vi "IPC-Core-ModbusModule.vi"(8 "error in":errorcluster, 9 "ErrorQRef":refnum<queue>, 10 "ModbusQRef":refnum<queue>, 11 "CmdQRef":refnum<queue>) -> (0 "error out":errorcluster)   [LabVIEW 2014]
uses:
  Configuration-Global.vi
panel:
  out "Modbus停止响应器":refnum<notifier>
  out "Modbus停止通知器":refnum<notifier>
  out "Modbus开始响应器":refnum<notifier>
  out "Modbus开始通知器":refnum<notifier>
  out "Modbus Deamo is Running":bool
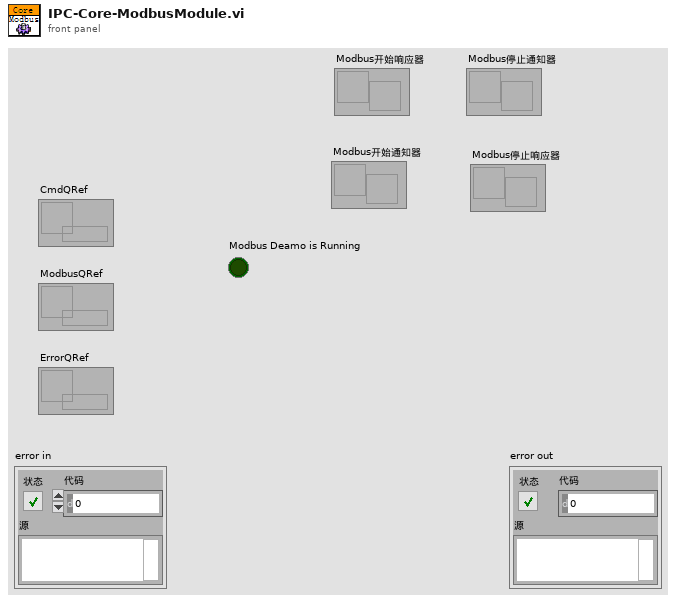
[diagram p1: front panel]
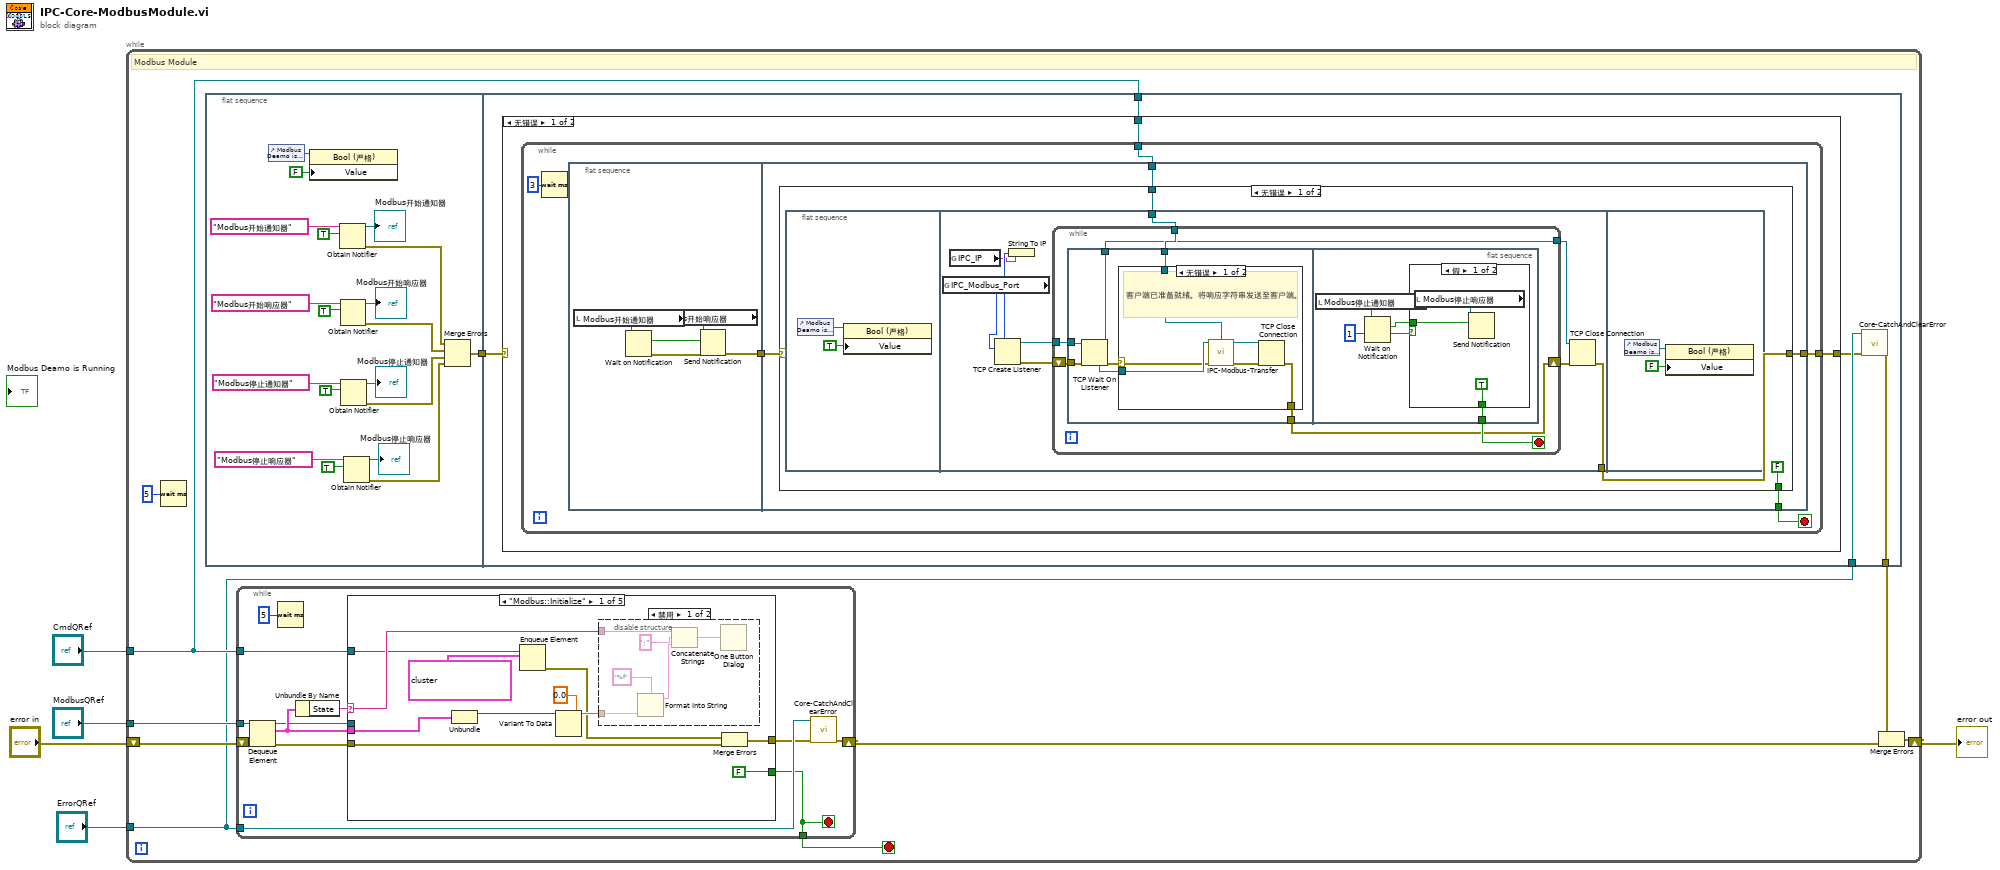
[diagram p0: block diagram]
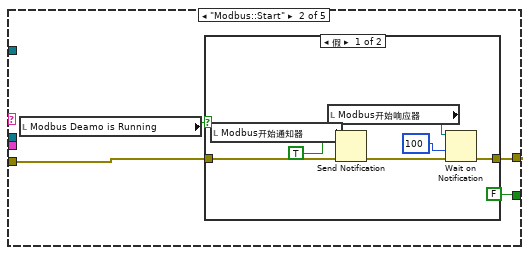
[diagram p3: hidden frame]
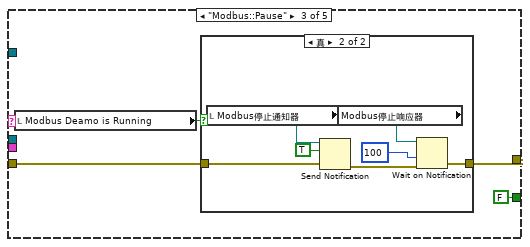
[diagram p5: hidden frame]
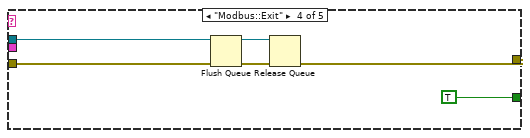
[diagram p7: hidden frame]
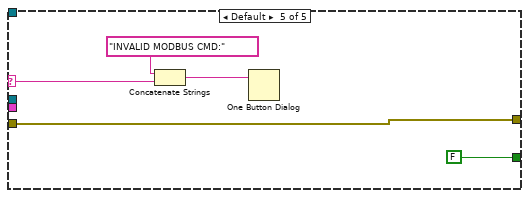
[diagram p8: hidden frame]
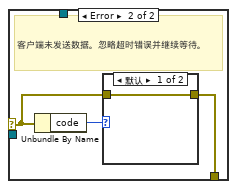
[diagram p9: hidden frame]
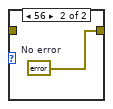
[diagram p10: hidden frame]
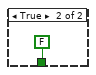
[diagram p11: hidden frame]
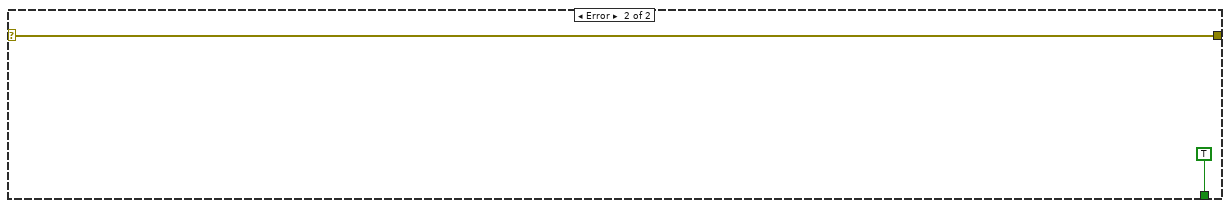
[diagram p12: hidden frame]
diagram:
  n1 = while {
    shift-right: [w6] -> w2
    shift-left: "error in" -> [w10]
    tunnel: "ErrorQRef" -> [w9]
    tunnel: "ModbusQRef" -> [w14]
    tunnel: "CmdQRef" -> [w11]
    stop <- w13 stop-if-true
    # "Modbus Module"
    n2 = Wait (ms)(milliseconds to wait=u32 5 ("等待时间（毫秒）")) -> ()  [unwired: 1 out]
    n3 = flat-sequence {
      tunnel: [w80] -> w12
      tunnel: w12 -> [w103]
      tunnel: w11 -> [w102]
      tunnel: w9 -> [w101]
      tunnel: [w99] -> w7
      frame #0 {
        n4 = control-ref of="Modbus Deamo is Running"() -> (w97:refnum<vi>)
        n5 = property class="Bool (严格)"(reference=w97, "Value"=FALSE ("值")) -> ()  [unwired: 1 in, 2 out]
        n6 = Obtain Notifier(name (unnamed)="Modbus开始通知器" ("名称（未命名）"), notification data type=TRUE) -> (notifier out=→"Modbus开始通知器":refnum<notifier>, error out=w84:errorcluster)  [unwired: 2 in, 1 out]
        n7 = Obtain Notifier(name (unnamed)="Modbus开始响应器" ("名称（未命名）"), notification data type=TRUE) -> (notifier out=→"Modbus开始响应器":refnum<notifier>, error out=w83:errorcluster)  [unwired: 2 in, 1 out]
        n8 = Obtain Notifier(name (unnamed)="Modbus停止通知器" ("名称（未命名）"), notification data type=TRUE) -> (notifier out=→"Modbus停止通知器":refnum<notifier>, error out=w82:errorcluster)  [unwired: 2 in, 1 out]
        n9 = Obtain Notifier(name (unnamed)="Modbus停止响应器" ("名称（未命名）"), notification data type=TRUE) -> (notifier out=→"Modbus停止响应器":refnum<notifier>, error out=w81:errorcluster)  [unwired: 2 in, 1 out]
        n10 = Merge Errors(w84, w83, w82, w81) -> (w80:errorcluster)
      }
      frame #1 {
        n11 = case shown="无错误" w103 {
          selector: w103 -> [_ w171]
          tunnel: w102 -> [w105 _]
          tunnel: [w104 w171] -> w100
          frame No Error {
            n12 = while {
              tunnel: w105 -> [w108]
              tunnel: [w107] -> w104
              stop <- w109 stop-if-true
              n13 = Wait (ms)(milliseconds to wait=u32 3 ("等待时间（毫秒）")) -> ()  [unwired: 1 out]
              n14 = flat-sequence {
                tunnel: [w111] -> w110
                tunnel: w110 -> [w119]
                tunnel: [w118] -> w109
                tunnel: w108 -> [w117]
                tunnel: [w116] -> w107
                frame #0 {
                  n15 = local read "Modbus开始通知器"() -> (w115:refnum<notifier>)
                  n16 = Wait on Notification(notifier=w115) -> (notification=w112:bool, error out=w113:errorcluster)  [unwired: 3 in, 2 out]
                  n17 = local read "Modbus开始响应器"() -> (w114:refnum<notifier>)
                  n18 = Send Notification(notification=w112, notifier=w114, error in (no error)=w113) -> (error out=w111:errorcluster)  [unwired: 1 out]
                }
                frame #1 {
                  n19 = case shown="无错误" w119 {
                    selector: w119 -> [_ w169]
                    tunnel: [FALSE TRUE] -> w118
                    tunnel: w117 -> [w121 _]
                    tunnel: [w120 w169] -> w116
                    frame No Error {
                      n20 = flat-sequence {
                        tunnel: w121 -> [w133]
                        tunnel: [w131] -> w120
                        frame #0 {
                          n21 = control-ref of="Modbus Deamo is Running"() -> (w123:refnum<vi>)
                          n22 = property class="Bool (严格)"(reference=w123, "Value"=TRUE ("值")) -> ()  [unwired: 1 in, 2 out]
                        }
                        frame #1 {
                          n23 = global read "Configuration-Global.vi" "IPC_Modbus_Port"() -> (w127:i32)
                          n24 = global read "Configuration-Global.vi" "IPC_IP"() -> (w125:string)
                          n25 = String To IP(1:w125) -> (0:w126:u32)
                          n26 = TCP Create Listener(7:w126, 10:w127) -> (0:w128:errorcluster, 3:w129:refnum<k5>)  [unwired: 3 in, 1 out]
                          n27 = while {
                            tunnel: w133 -> [w138]
                            tunnel: w129 -> [w137]
                            tunnel: [w135] -> w132
                            shift-right: [w134] -> w130
                            shift-left: w128 -> [w136]
                            stop <- w139 stop-if-true
                            n28 = flat-sequence {
                              tunnel: w138 -> [w146]
                              tunnel: w137 -> [w145]
                              tunnel: w136 -> [w144]
                              tunnel: [w143] -> w135
                              tunnel: [w141] -> w134
                              tunnel: [w162] -> w139
                              frame #0 {
                                n29 = TCP Wait On Listener(8:w144, 11:w145) -> (0:w140:errorcluster, 3:w143:refnum<k5>, 4:w142:refnum<k5>)  [unwired: 2 in, 2 out]
                                n30 = case shown="无错误" w140 {
                                selector: w140 -> [w147 w154]
                                tunnel: w146 -> [w152 _]
                                tunnel: w142 -> [w151 _]
                                tunnel: [w148 w153] -> w141
                                frame No Error {
                                # "客户端已准备就绪。将响应字符串发送至客户端。"
                                n31 = call "IPC-Modbus-Transfer.vi"("connection ID in"=w151, "CmdQRef"=w152, "错误输入（无错误）"=w147) -> ("connection ID out"=w150:refnum<k5>, "错误输出"=w149:errorcluster)  [unwired: 11 in]
                                n32 = TCP Close Connection(connection ID=w150, error in (no error)=w149) -> (error out=w148:errorcluster)  [unwired: 1 in, 1 out]
                                }
                                frame Error {
                                # "客户端未发送数据。忽略超时错误并继续等待。"
                                n33 = Unbundle By Name(w154) -> ("code"=w155:i32)
                                n34 = case shown="默认" w155 {
                                tunnel: w154 -> [w156 _]
                                tunnel: [w156 w157] -> w153
                                frame Default {
                                }
                                frame 56 {
                                w157 = errorcluster {"status"=FALSE, "code"=0, "source"=""}  # No error
                                }
                                }
                                }
                                }
                              }
                              frame #1 {
                                n35 = local read "Modbus停止通知器"() -> (w160:refnum<notifier>)
                                n36 = Wait on Notification(notifier=w160, timeout in ms (-1)=1 ("超时毫秒(-1)")) -> (notification=w158:bool, timed out?=w159:bool)  [unwired: 2 in, 2 out]
                                n37 = case shown="假" w159 {
                                tunnel: [TRUE FALSE] -> w162
                                tunnel: w158 -> [w164 _]
                                frame False {
                                n38 = local read "Modbus停止响应器"() -> (w163:refnum<notifier>)
                                n39 = Send Notification(notification=w164, notifier=w163) -> ()  [unwired: 1 in, 2 out]
                                }
                                frame True {
                                }
                                }
                              }
                            }
                          }
                          n40 = TCP Close Connection(connection ID=w132, error in (no error)=w130) -> (error out=w131:errorcluster)  [unwired: 1 in, 1 out]
                        }
                        frame #2 {
                          n41 = control-ref of="Modbus Deamo is Running"() -> (w167:refnum<vi>)
                          n42 = property class="Bool (严格)"(reference=w167, "Value"=FALSE ("值")) -> ()  [unwired: 1 in, 2 out]
                        }
                      }
                    }
                    frame Error {
                    }
                  }
                }
              }
            }
          }
          frame Error {
          }
        }
        n43 = call "Core-CatchAndClearError.vi"("error in (no error)"=w100, "ErrorQ"=w101) -> ("error out"=w99:errorcluster)  [unwired: 7 in]
      }
    }
    n44 = while {
      tunnel: w9 -> [w23]
      tunnel: w14 -> [w20]
      tunnel: [w17] -> w13
      tunnel: w11 -> [w18]
      shift-right: [w24] -> w8
      shift-left: w10 -> [w27]
      stop <- w17 stop-if-true
      n45 = Dequeue Element(queue=w20, error in (no error)=w27) -> (queue out=w19:refnum<queue>, element=w21:cluster{"Data":variant, "State":string}, error out=w26:errorcluster)  [unwired: 1 in, 1 out]
      n46 = Wait (ms)(milliseconds to wait=u32 5 ("等待时间（毫秒）")) -> ()  [unwired: 1 out]
      n47 = Unbundle By Name(w21) -> ("State"=w25:string)
      n48 = case shown="\"Modbus::Initialize\"" w25 {
        selector: w25 -> [w34 _ _ _ w76]
        tunnel: w26 -> [w29 w47 w59 w71 w79]
        tunnel: [w28 w48 w58 w72 w79] -> w22
        tunnel: w21 -> [w38 _ _ _ _]
        tunnel: w19 -> [_ _ _ w70 _]
        tunnel: [FALSE FALSE FALSE TRUE FALSE] -> w17
        tunnel: w18 -> [w32 _ _ _ _]
        frame "Modbus::Initialize" {
          n49 = Unbundle(w38) -> ("Data"=w37:variant)  [unwired: 1 out]
          n50 = Enqueue Element(queue=w32, element=cluster{"Data":variant, "State":string} {"Data"=variant, "State"="Cmd::StartModbus"} ("元素")) -> (error out=w30:errorcluster)  [unwired: 2 in, 2 out]
          n51 = Variant To Data(type=0.0, Variant=w37) -> (data=w33:dbl)  [unwired: 1 in, 1 out]
          n52 = disable-structure shown="禁用" {
            disable-tunnel: w34 -> [w44 _]
            disable-tunnel: w33 -> [w41 _]
            frame Disabled {
              n53 = Format Into String(format string="%f" ("格式字符串"), w41) -> (resulting string=w40:string)  [unwired: 2 in, 1 out]
              n54 = Concatenate Strings(w44, ":" ("字符串"), w40) -> (w43:string)
              n55 = One Button Dialog(message=w43) -> ()  [unwired: 1 in, 1 out]
            }
            frame Enabled {
            }
          }
          n56 = Merge Errors(w30, w29) -> (w28:errorcluster)
        }
        frame "Modbus::Start" {
          n57 = local read "Modbus Deamo is Running"() -> (w45:bool)
          n58 = case shown="假" w45 {
            tunnel: [w50 w56] -> w48
            tunnel: w47 -> [w49 w56]
            frame False {
              n59 = local read "Modbus开始通知器"() -> (w55:refnum<notifier>)
              n60 = local read "Modbus开始响应器"() -> (w52:refnum<notifier>)
              n61 = Send Notification(notification=TRUE ("通知"), notifier=w55, error in (no error)=w49) -> (error out=w53:errorcluster)  [unwired: 1 out]
              n62 = Wait on Notification(notifier=w52, timeout in ms (-1)=100 ("超时毫秒(-1)"), error in (no error)=w53) -> (error out=w50:errorcluster)  [unwired: 1 in, 3 out]
            }
            frame True {
            }
          }
        }
        frame "Modbus::Pause" {
          n63 = local read "Modbus Deamo is Running"() -> (w60:bool)
          n64 = case shown="真" w60 {
            tunnel: w59 -> [w61 w64]
            tunnel: [w61 w65] -> w58
            frame False {
            }
            frame True {
              n65 = local read "Modbus停止通知器"() -> (w68:refnum<notifier>)
              n66 = Send Notification(notification=TRUE ("通知"), notifier=w68, error in (no error)=w64) -> (error out=w66:errorcluster)  [unwired: 1 out]
              n67 = local read "Modbus停止响应器"() -> (w67:refnum<notifier>)
              n68 = Wait on Notification(notifier=w67, timeout in ms (-1)=100 ("超时毫秒(-1)"), error in (no error)=w66) -> (error out=w65:errorcluster)  [unwired: 1 in, 3 out]
            }
          }
        }
        frame "Modbus::Exit" {
          n69 = Flush Queue(queue=w70, error in (no error)=w71) -> (queue out=w74:refnum<queue>, error out=w73:errorcluster)  [unwired: 1 out]
          n70 = Release Queue(queue=w74, error in (no error)=w73) -> (error out=w72:errorcluster)  [unwired: 1 in, 2 out]
        }
        frame Default {
          n71 = Concatenate Strings("INVALID MODBUS CMD:", w76) -> (w77:string)
          n72 = One Button Dialog(message=w77) -> ()  [unwired: 1 in, 1 out]
        }
      }
      n73 = call "Core-CatchAndClearError.vi"("error in (no error)"=w22, "ErrorQ"=w23) -> ("error out"=w24:errorcluster)  [unwired: 7 in]
    }
    n74 = Merge Errors(w7, w8) -> (w6:errorcluster)
  }
  "error out" <- w2
